vi "RecordingPath.vi"(8 "error in (no error)":errorcluster, 9 "Extension":string, 10 "Recording Root":path=path "C:/", 11 "Electrophysiology in":refnum<class "Electrophysiology.lvclass">) -> (0 "error out":errorcluster, 2 "FilePath":path, 3 "Electrophysiology out":refnum<class "Electrophysiology.lvclass">)   [LabVIEW 2010]
uses:
  Electrophysiology.lvclass
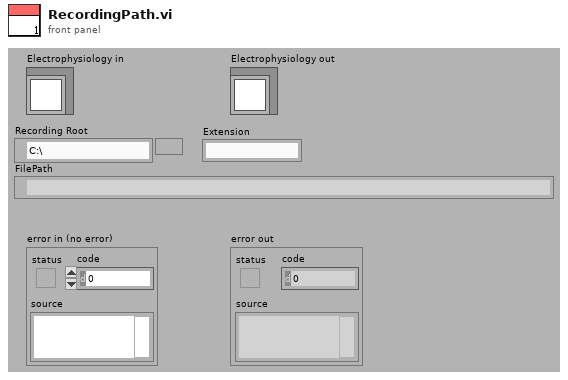
[diagram p1: front panel]
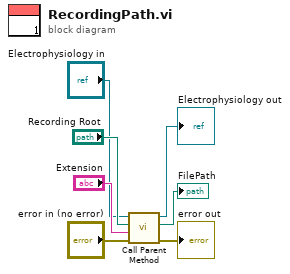
[diagram p0: block diagram]
diagram:
  n1 = call-parent "Call Parent Method"("error in (no error)"="error in (no error)", "Extension"="Extension", "Recording Root"="Recording Root", "AcquistionObject in"="Electrophysiology in") -> ("error out"=→"error out":errorcluster, "FilePath"=→"FilePath":path, "AcquistionObject out"=→"Electrophysiology out":refnum<class "Electrophysiology.lvclass">)  [unwired: 5 in]
